vi "Copy Firmware.vi"(2 "Error In":errorcluster, 3 "Copy Software Only":bool, 4 "Image Destination":T1, 5 "Image Source":T1) -> (0 "Error Out":errorcluster, 1 "Messages":string)   [LabVIEW 2018]
uses:
  Image Parameters.ctl
  Type Defs/State Machine.ctl
  Type Defs/Global Action.ctl
  Type Defs/Save Options.ctl
  Type Defs/RT Command.ctl
  Type Defs/Insrument State.ctl
  <vilib>/nisyscfg/Set System Image (Folder).vi
  <vilib>/nisyscfg/Close (System).vi
  <vilib>/nisyscfg/Create System Image (Folder).vi
  <vilib>/nisyscfg/nisyscfg.lvlib
panel:
  out "IP Address":string
  out "Current Task":string
  # "Please wait up to a few minutes while copying firmware"
  # "(This dialog will automatically close when update is finished)"
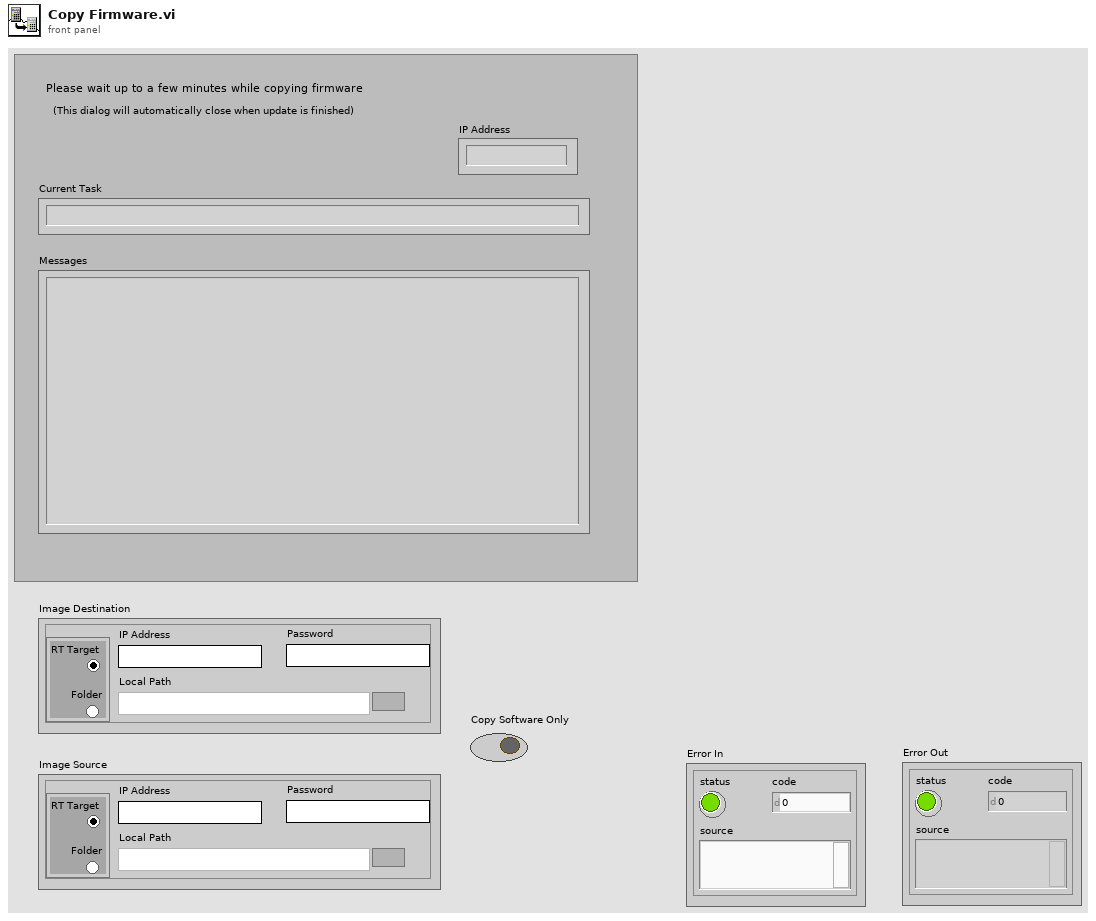
[diagram p1: front panel]
types:
  T1 = typedef "Image Parameters.ctl" = cluster{"Radio Buttons":enum32{"RT Target", "Folder"}, "Local Path":path, "IP Address":string, "Password ":string}
  T2 = typedef "State Machine.ctl" = enum16{"Wait", "Init", "Case 0", "Case 1", "Case 2", "Case 3", "Case 4", "Case 5", "Case 6", "Case 7", "Case 8", "Case 9", "Case 10", "Error", "Exit"}
  T3 = typedef "Global Action.ctl" = enum16{"Write", "Read"}
  T4 = typedef "Save Options.ctl" = enum16{"Use Dialog", "Temporary File", "My Tables", "Full Path"}
  T5 = typedef "RT Command.ctl" = enum16{"xml Start Run", "xml Start Actual Run", "xml Stop Run", "xml Runtime Update", "xml Get Status", "xml Get Table", "xml Set Table", "xml Get Configuration", "xml System Status", "xml Set LC Input Logic", "xml Get Data", "xml Get Info", "Start", "StartActualRun", "Stop", "Runtime Update", "Get Data", "Get Info", "Get Status", "Get Param", "Get Config", "Get Table", "Read ADC", "Set Oscillator", "Update Config", "Update Table", "Set All Pol", "Set Pol and DC", "Set Max Mass", "Toggle RP", "Toggle EL", "Set PIC", "Initialize Turbo", "Send Turbo Comm", "Close Turbo", "P1", "P2", "P3", "Send Serial", "Set LC Out", "Get LC In", "Read VAC", "Test Table", "Toggle Power", "Get Startup", "Set Startup", "Get ADC Table", "Set ADC Table", "Get Brief Status", "Get Detail Status", "Auxiliary Update", "Set CC Logics", "Set CC Input Logics", "Ignore Error", "invalid"}
  T6 = typedef "Insrument State.ctl" = enum16{"Initializing", "Mass Spectrometer is Off", "Starting Up", "Turning Power Off", "Going to Standby", "Roughing Pump Ready", "Turning Turbo Off", "Turbo Startup", "Turbopump Ready", "Checking Vacuum", "Going to Ready", "Ready", "Running", "Source Standby", "Lost Communication", "Shutting Down", "Fault", "24V Standby", "Go to 24V Standby", "Turbopump Ready-Waiting"}
  T7 = typedef "Global Configrations.ctl" = cluster{"Model Name":enum16{"QSight 110", "QSight 120", "QSight 210", "QSight 220", "QSight 410", "QSight 420", "IONICS 3Q 110", "IONICS 3Q 120", "IONICS 3Q 210", "IONICS 3Q 220", "IONICS 3Q 310", "IONICS 3Q 320", "Simulation (Single Source)", "Simulation (Dual Source)"}, "RunType":u16, "Acquisition State":enum16{"Ready", "Busy", "Waiting"}, "InstrState":enum16{"Initializing", "Mass Spectrometer is Off", "Starting Up", "Turning Power Off", "Going to Standby", "Roughing Pump Ready", "Turning Turbo Off", "Turbo Startup", "Turbopump Ready", "Checking Vacuum", "Going to Ready", "Ready", "Running", "Source Standby", "Lost Communication", "Shutting Down", "Fault", "24V Standby", "Go to 24V Standby", "Turbopump Ready-Waiting"}, "Run Mode":enum16{"MRM (Q1/Q2)", "Q1 Scan", "Q1 SRM", "Q2 Scan", "Q2 SRM", "Product Scan", "Precursor Scan", "Neutral Loss", "Neutral Gain"}, "Configration":T8, "TCP ID":refnum<k5>, "DT":bool, "Dead Time (nS)":i32, "Single Source":bool, "ADC Tables":T10[], "FW Udate":bool, "Simulator":bool}
  T8 = typedef "Configration.ctl" = cluster{"Table":T9[], "Instrument":string[]}
  T9 = typedef "_RT Configuration 2.ctl" = cluster{"Name":string, "Ch#":u8, "Min":dbl, "Max":dbl, "Def+":dbl, "Def-":dbl, "Offset":dbl, "Slope":dbl, "Type":u8, "Description":string, "SettleT":dbl}
  T10 = typedef "ADC Table.ctl" = cluster{"Name":string, "Ch#":u8, "Min":dbl, "Max":dbl, "Def+":dbl, "Def-":dbl, "Offset":dbl, "Slope":dbl, "Type":u8, "Description":string, "SettleT":dbl}
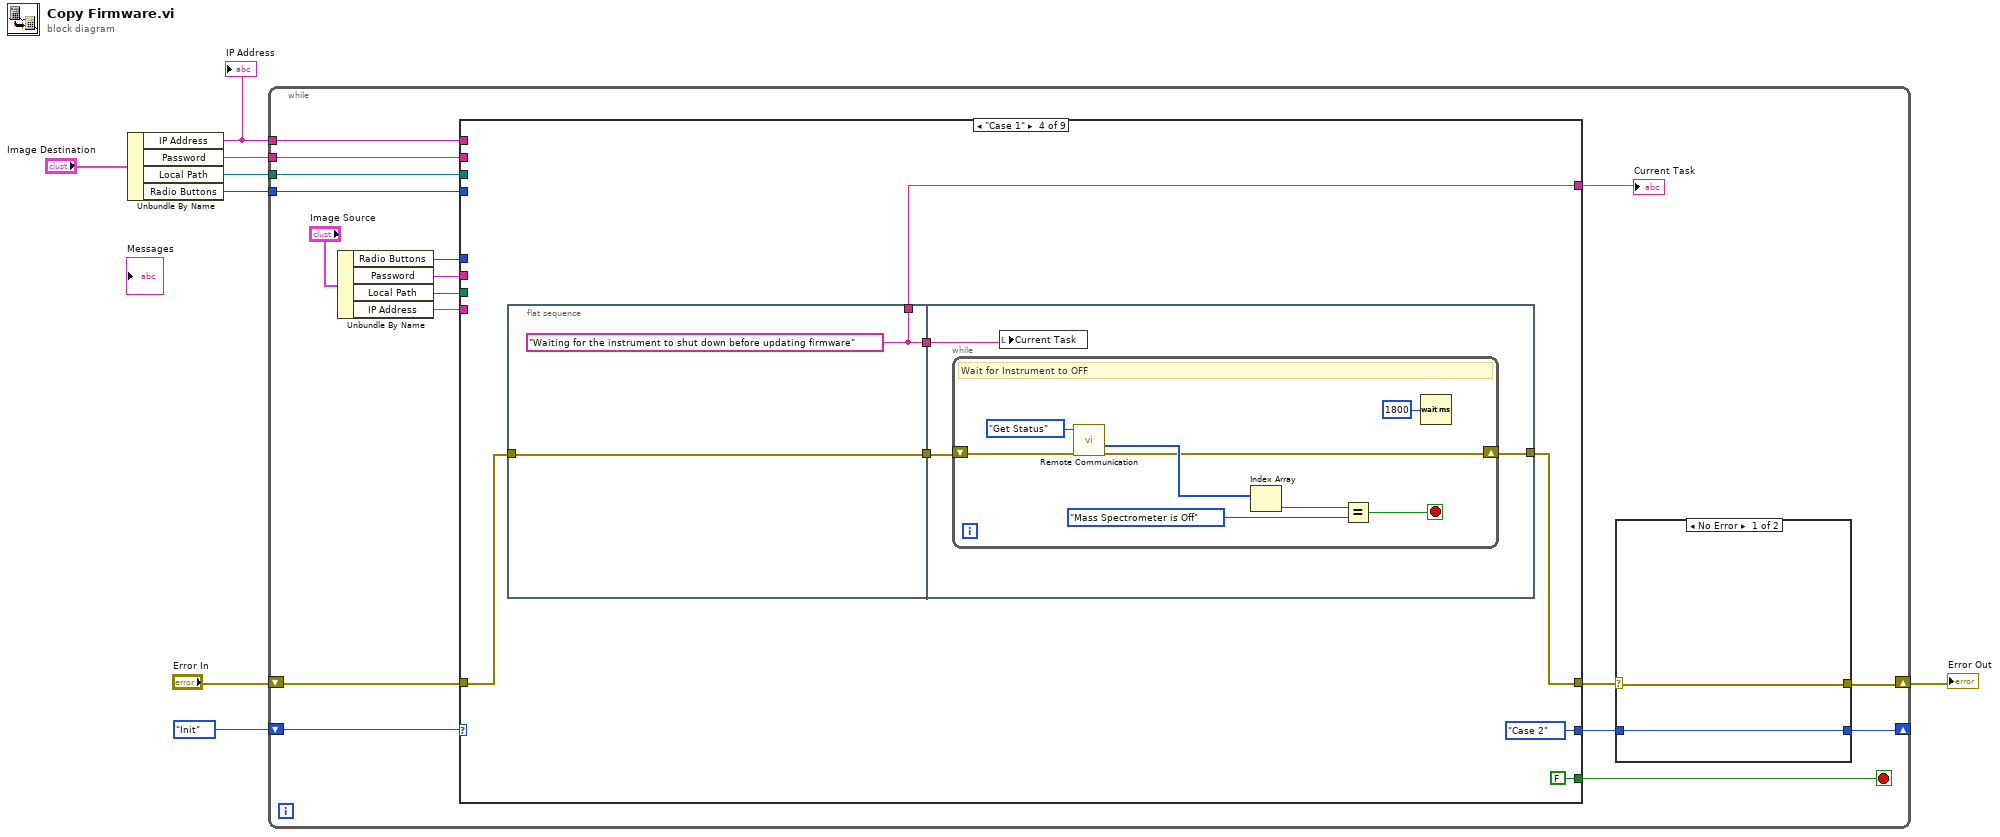
[diagram p0: block diagram]
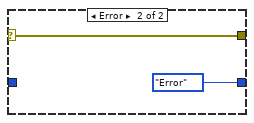
[diagram p2: hidden frame]
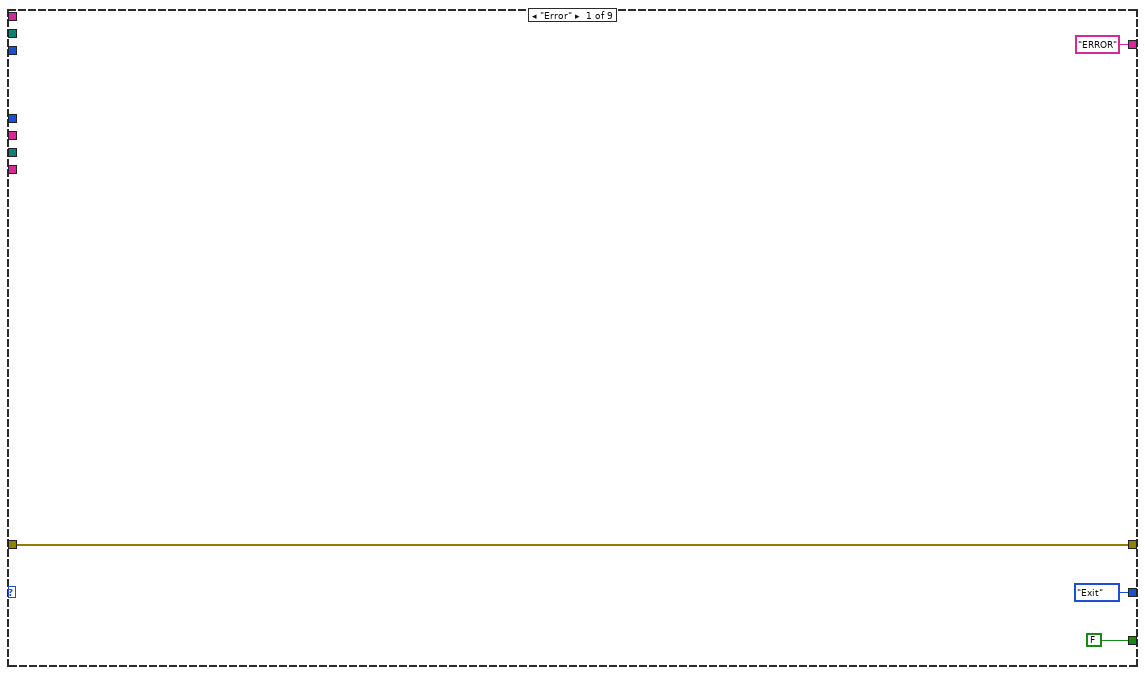
[diagram p3: hidden frame]
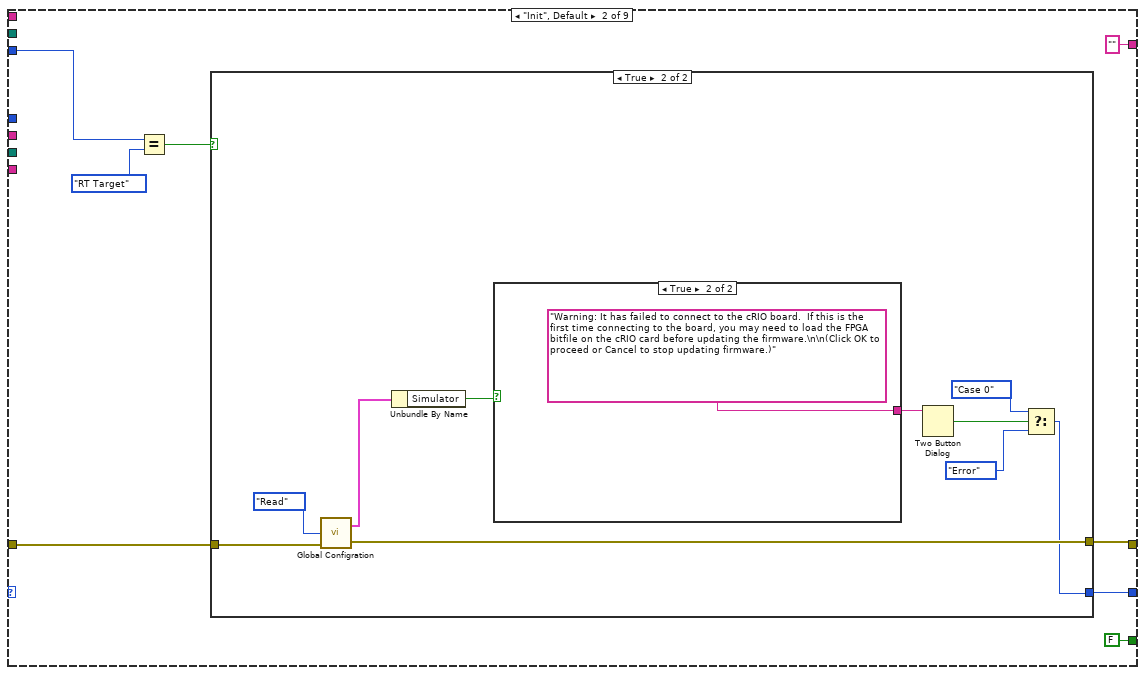
[diagram p4: hidden frame]
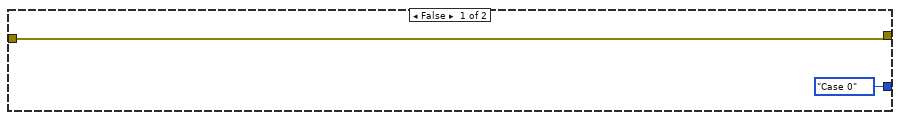
[diagram p5: hidden frame]
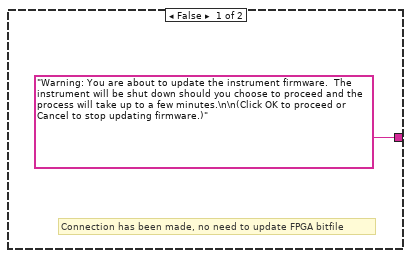
[diagram p6: hidden frame]
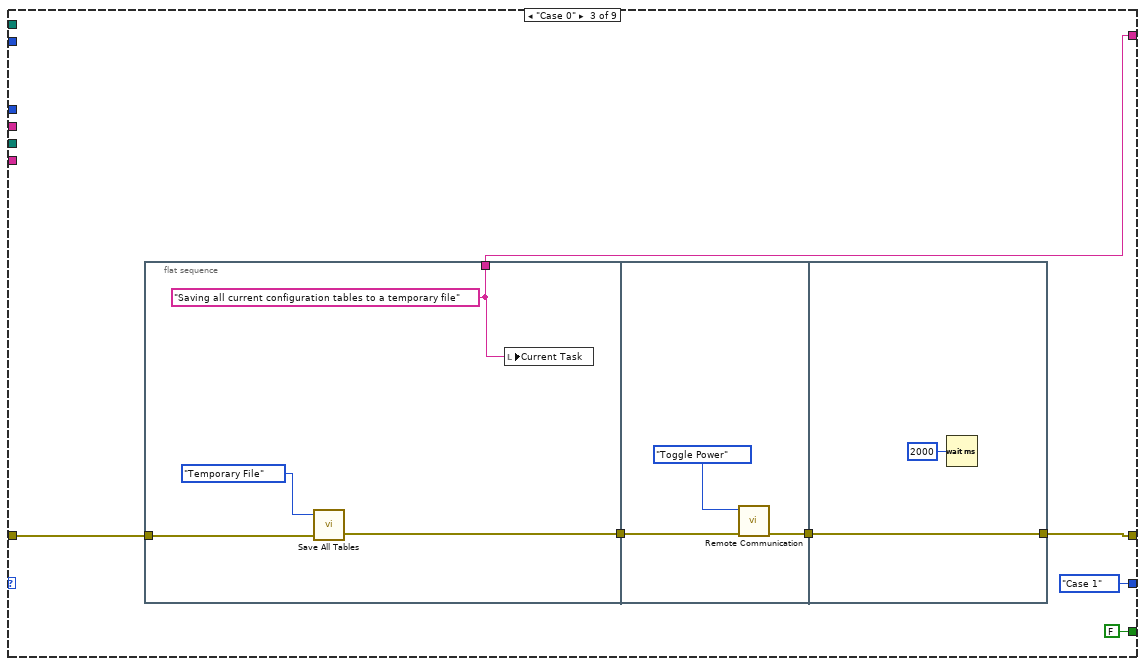
[diagram p7: hidden frame]
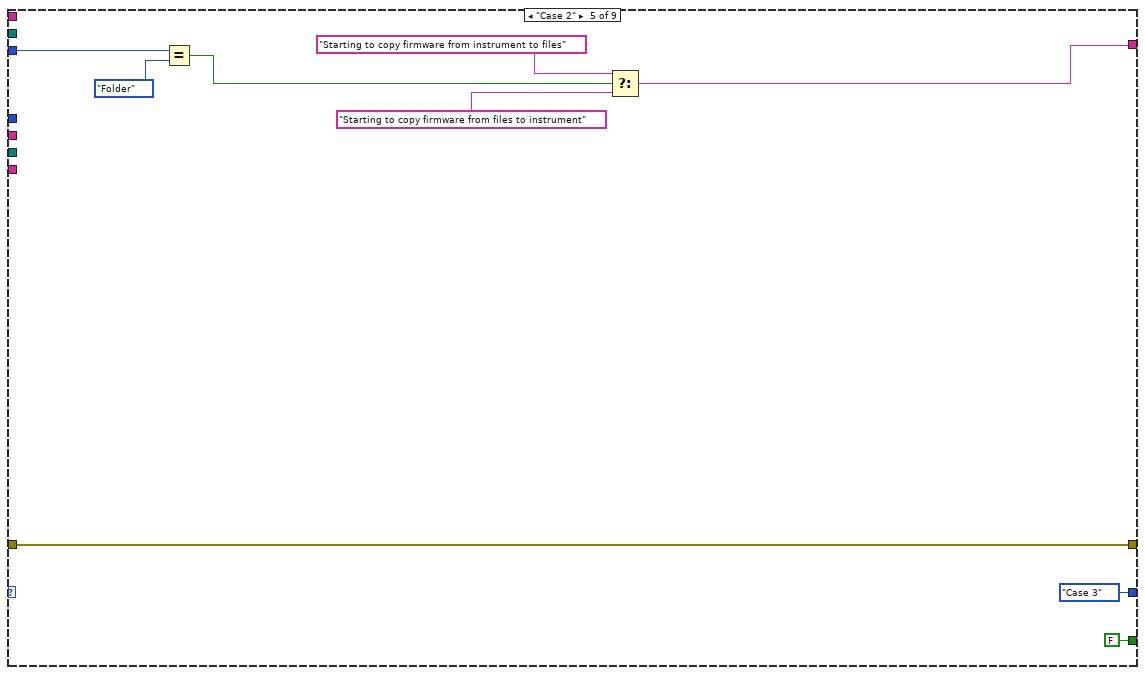
[diagram p8: hidden frame]
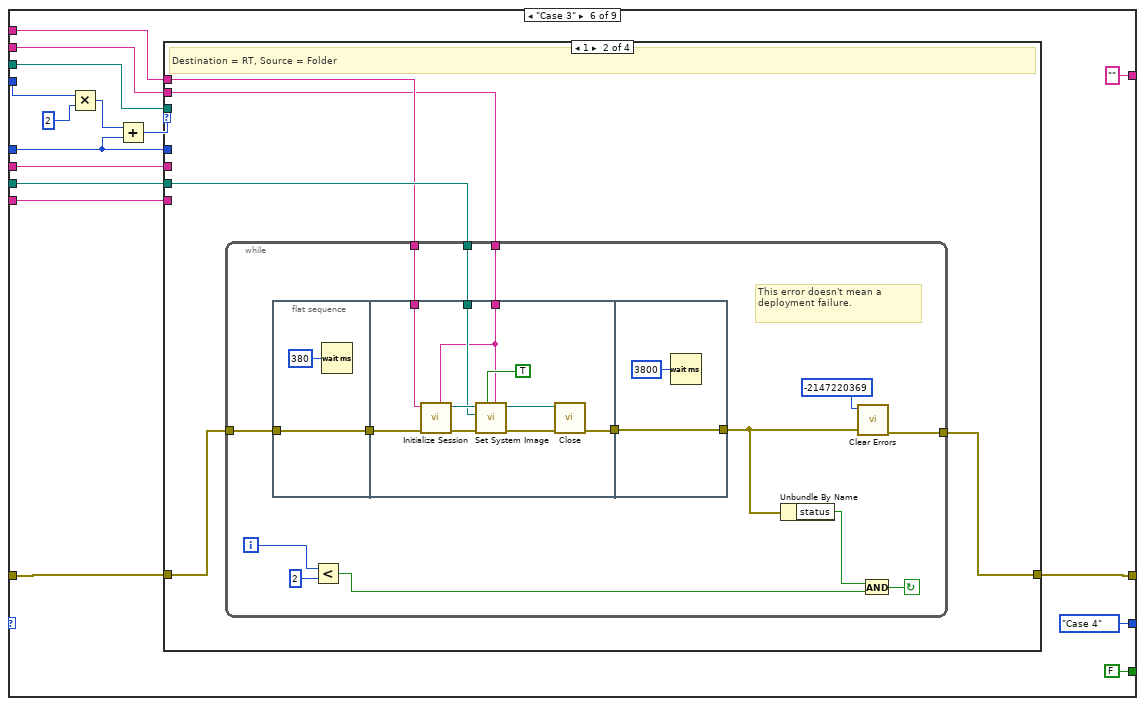
[diagram p9: hidden frame]
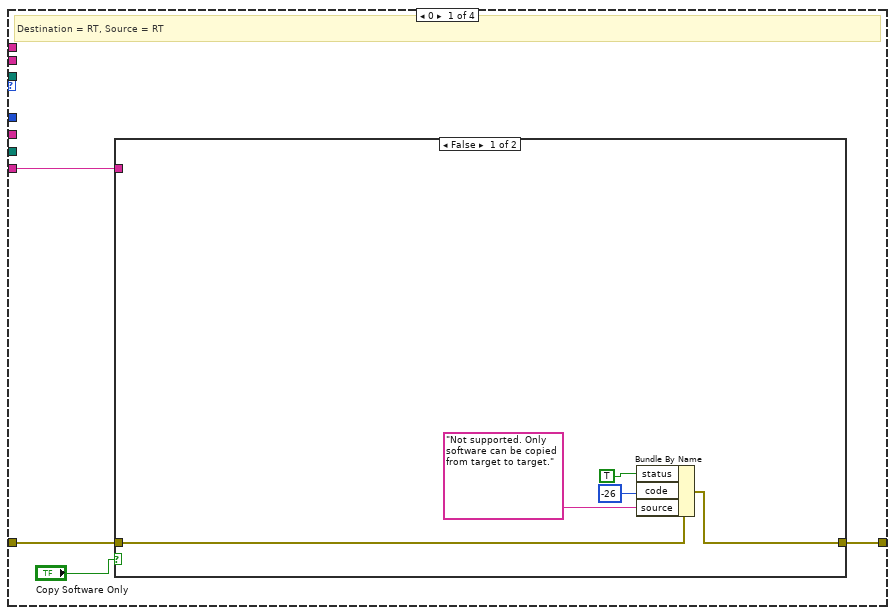
[diagram p10: hidden frame]
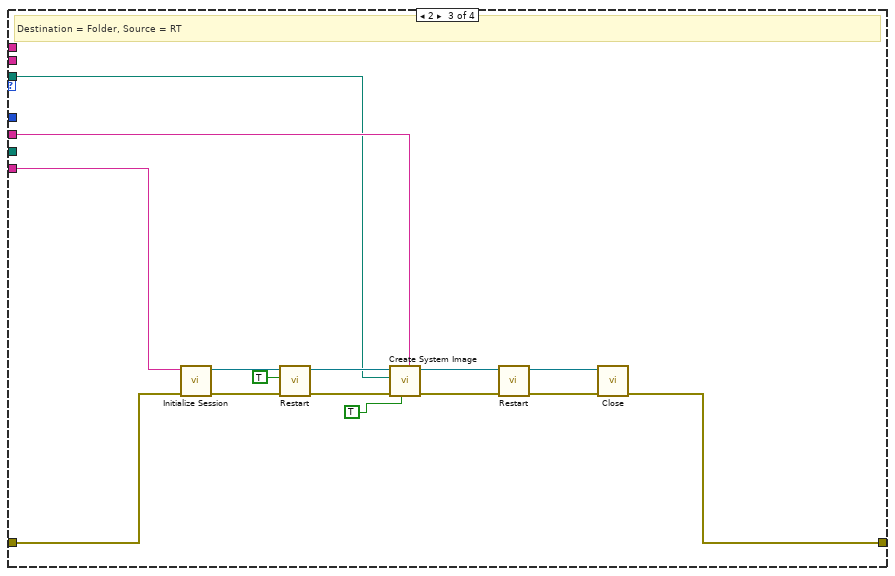
[diagram p12: hidden frame]
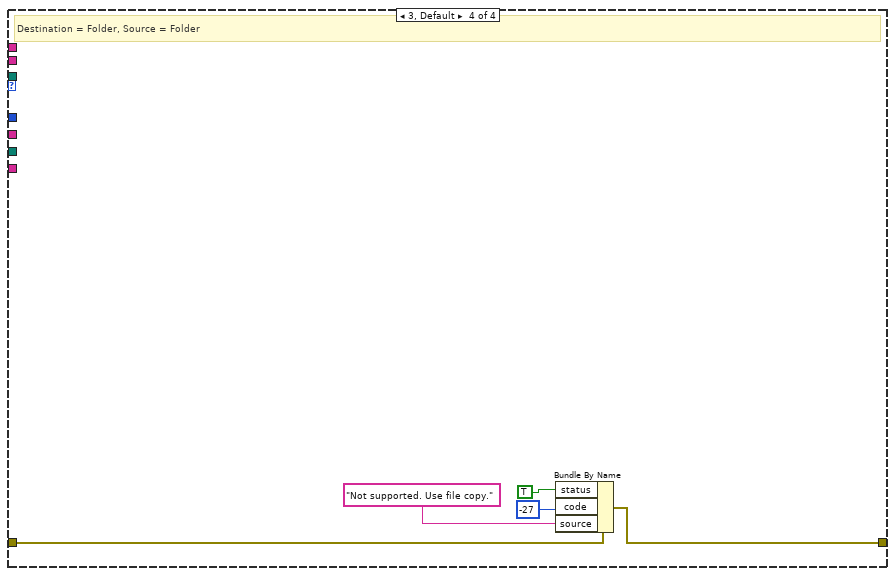
[diagram p13: hidden frame]
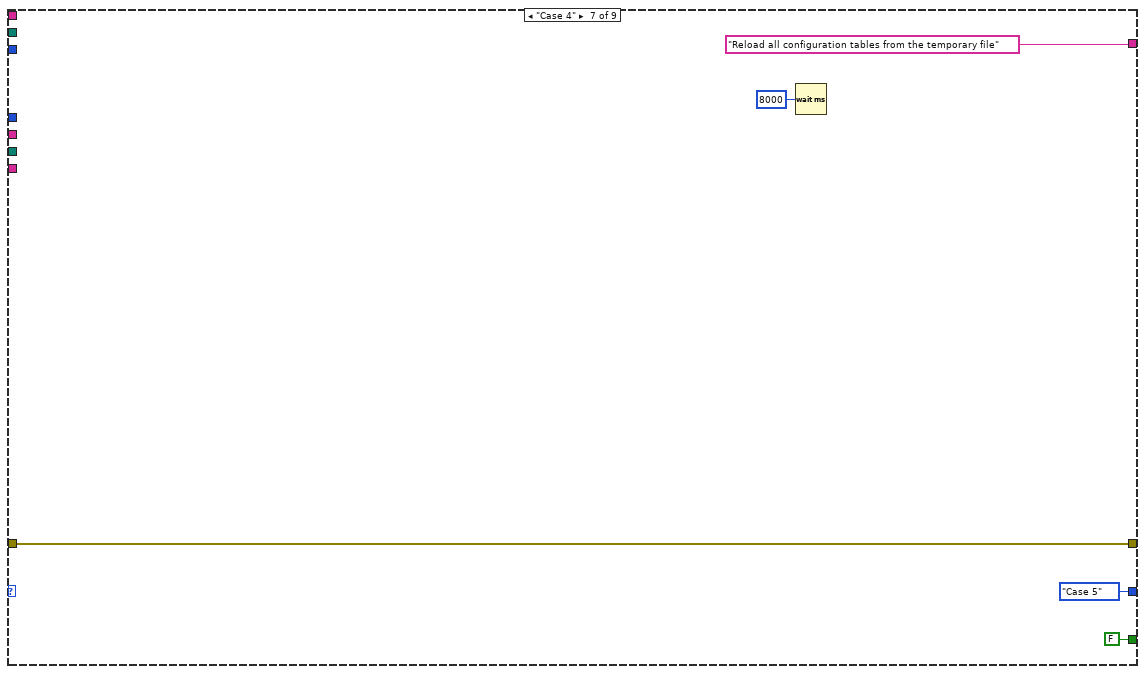
[diagram p14: hidden frame]
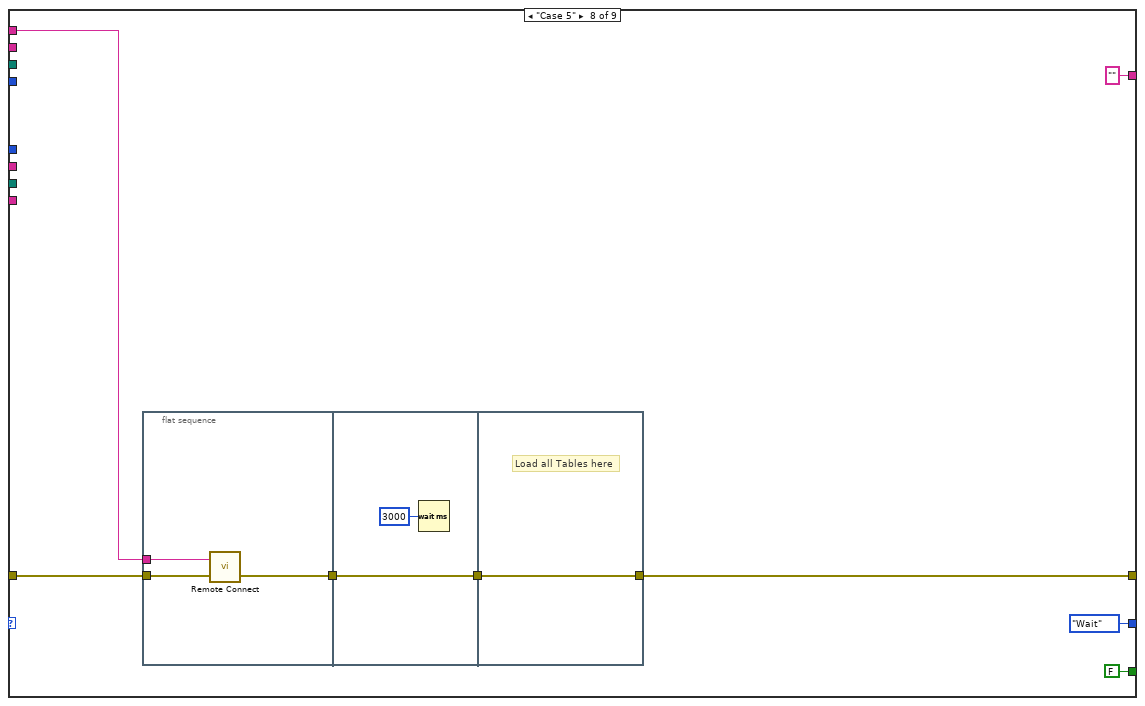
[diagram p15: hidden frame]
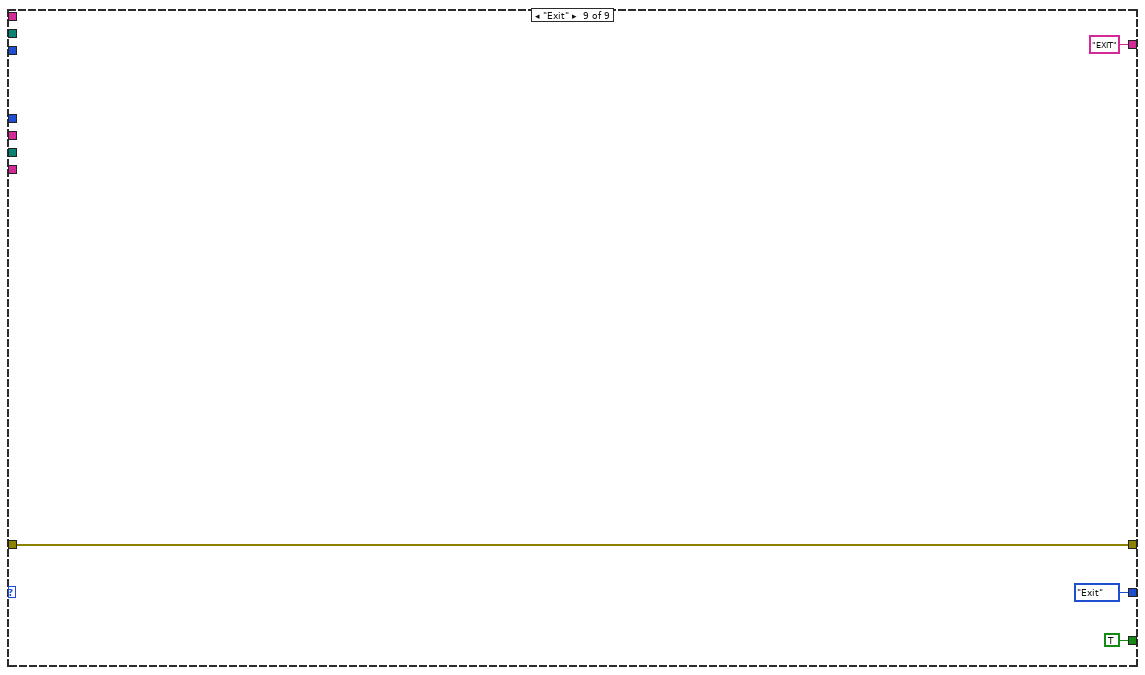
[diagram p16: hidden frame]
diagram:
  n1 = Unbundle By Name("Image Destination") -> ("IP Address"=w4:string, "Password"=w3:string, "Local Path"=w2:path, "Radio Buttons"=w1:enum32{"RT Target", "Folder"})
  "IP Address" <- w4
  n2 = while {
    shift-right: [w22] -> _
    shift-left: State_Machine."Init" ("Enum") -> [w25]
    shift-right: [w18] -> w6
    shift-left: "Error In" -> [w24]
    tunnel: w4 -> [w17]
    tunnel: w3 -> [w16]
    tunnel: w2 -> [w10]
    tunnel: w1 -> [w20]
    stop <- w9 stop-if-true
    n3 = Unbundle By Name("Image Source") -> ("Radio Buttons"=w14:enum32{"RT Target", "Folder"}, "Password"=w13:string, "Local Path"=w12:path, "IP Address"=w11:string)
    n4 = case shown="\"Case 1\"" w25 {
      tunnel: w24 -> [w30 w36 w60 w74 w94 w112 w180 w192 w200]
      tunnel: [w30 w35 w56 w73 w94 w111 w180 w188 w200] -> w23
      tunnel: [State_Machine."Exit" ("Enum") w34 State_Machine."Case 1" ("Enum") State_Machine."Case 2" ("Enum") State_Machine."Case 3" ("Enum") State_Machine."Case 4" ("Enum") State_Machine."Case 5" ("Enum") State_Machine."Wait" ("Enum") State_Machine."Exit" ("Enum")] -> w21
      tunnel: [FALSE FALSE FALSE FALSE FALSE FALSE FALSE FALSE TRUE] -> w9
      tunnel: w20 -> [_ w40 _ _ w100 w116 _ _ _]
      tunnel: ["ERROR" "" w57 w76 w95 "" "Reload all configuration tables from the temporary file" "" "EXIT"] -> w19
      tunnel: w17 -> [_ _ _ _ _ w106 _ w191 _]
      tunnel: w16 -> [_ _ _ _ _ w105 _ _ _]
      tunnel: w14 -> [_ _ _ _ _ w107 _ _ _]
      tunnel: w13 -> [_ _ _ _ _ w110 _ _ _]
      tunnel: w12 -> [_ _ _ _ _ w108 _ _ _]
      tunnel: w11 -> [_ _ _ _ _ w109 _ _ _]
      tunnel: w10 -> [_ _ _ _ _ w102 _ _ _]
      frame "Error" {
      }
      frame "Init", Default {
        n5 = Equal?(x=w40, y=enum32{"RT Target", "Folder"}."RT Target") -> (x = y?=w37:bool)
        n6 = case shown="True" w37 {
          tunnel: w36 -> [w43 w52]
          tunnel: [w43 w48] -> w35
          tunnel: [State_Machine."Case 0" ("Enum") w47] -> w34
          frame False {
          }
          frame True {
            n7 = call "Global Configration.vi"("Error In"=w52, "Action"=Global_Action."Read") -> ("Error Out"=w48:errorcluster, "Parameters Out"=w50:T7)  [unwired: 1 in]
            n8 = Unbundle By Name(w50) -> ("Simulator"=w49:bool)
            n9 = case shown="True" w49 {
              tunnel: ["Warning: You are about to update the instrument firmware.  The instrument will be shut down should you choose to proceed and the process will take up to a few minutes.\n\n(Click OK to proceed or Cancel to stop updating firmware.)" "Warning: It has failed to connect to the cRIO board.  If this is the first time connecting to the board, you may need to load the FPGA bitfile on the cRIO card before updating the firmware.\n\n(Click OK to proceed or Cancel to stop updating firmware.)"] -> w53
              frame False {
                # "Connection has been made, no need to update FPGA bitfile"
              }
              frame True {
              }
            }
            n10 = Two Button Dialog(message=w53) -> (T button?=w44:bool)  [unwired: 2 out]
            n11 = Select(t=State_Machine."Case 0" ("Enum"), s=w44, f=State_Machine."Error" ("Enum")) -> (s? t:f=w47:T2)
          }
        }
      }
      frame "Case 0" {
        n12 = flat-sequence {
          tunnel: w60 -> [w65]
          tunnel: [w64] -> w59
          tunnel: [w63] -> w57
          tunnel: w59 -> [w68]
          tunnel: [w67] -> w58
          tunnel: [w71] -> w56
          tunnel: w58 -> [w71]
          frame #0 {
            w63 = "Saving all current configuration tables to a temporary file"
            n13 = call "Save All Tables.vi"("Error In"=w65, "SaveOption(Temporary File)"=Save_Options."Temporary File") -> ("Error Out"=w64:errorcluster)  [unwired: 1 in, 1 out]
            n14 = local write "Current Task"(w63) -> ()
          }
          frame #1 {
            n15 = call "Remote Communication.vi"("Error In"=w68, "Command"=RT_Command."Toggle Power") -> ("Error Out"=w67:errorcluster)  [unwired: 4 in, 3 out]
          }
          frame #2 {
            n16 = Wait (ms)(milliseconds to wait=u32 2000) -> ()  [unwired: 1 out]
          }
        }
      }
      frame "Case 1" {
        n17 = flat-sequence {
          tunnel: [w79] -> w76
          tunnel: [w80] -> w75
          tunnel: w74 -> [w80]
          tunnel: [w79] -> w72
          tunnel: w75 -> [w83]
          tunnel: [w82] -> w73
          tunnel: w72 -> [w81]
          frame #0 {
            w79 = "Waiting for the instrument to shut down before updating firmware"
          }
          frame #1 {
            n18 = while {
              shift-right: [w86] -> w82
              shift-left: w83 -> [w85]
              stop <- w87 stop-if-true
              # "Wait for Instrument to OFF"
              n19 = call "Remote Communication.vi"("Error In"=w85, "Command"=RT_Command."Get Status") -> ("Error Out"=w86:errorcluster, "Data Array"=w90:i32[])  [unwired: 4 in, 2 out]
              n20 = Index Array(array=w90) -> (element=w91:i32)  [unwired: 1 in]
              n21 = Equal?(x=w91, y=Insrument_State."Mass Spectrometer is Off" ("InstrState")) -> (x = y?=w87:bool)
              n22 = Wait (ms)(milliseconds to wait=u32 1800) -> ()  [unwired: 1 out]
            }
            n23 = local write "Current Task"(w81) -> ()
          }
        }
      }
      frame "Case 2" {
        n24 = Equal?(x=w100, y=enum32{"RT Target", "Folder"}."Folder") -> (x = y?=w97:bool)
        n25 = Select(t="Starting to copy firmware from instrument to files", s=w97, f="Starting to copy firmware from files to instrument") -> (s? t:f=w95:string)
      }
      frame "Case 3" {
        n26 = Multiply(x=w116, y=2) -> (x*y=w114:u32)
        n27 = Add(x=w114, y=w107) -> (x+y=w113:u32)
        n28 = case shown="1" w113 {
          tunnel: w112 -> [w119 w131 w164 w176]
          tunnel: [w118 w127 w163 w175] -> w111
          tunnel: w110 -> [_ _ w162 _]
          tunnel: w109 -> [w117 _ w161 _]
          tunnel: w108 -> [_ w130 _ _]
          tunnel: w107 -> [_ _ _ _]
          tunnel: w106 -> [_ w129 _ _]
          tunnel: w105 -> [_ w128 _ _]
          tunnel: w102 -> [_ _ w160 _]
          frame 0 {
            # "Destination = RT, Source = RT"
            n29 = case shown="False" "Copy Software Only" {
              tunnel: w119 -> [w122 w126]
              tunnel: [w121 w126] -> w118
              tunnel: w117 -> [_ _]
              frame False {
                n30 = Bundle By Name(cluster=w122, "status"=TRUE, "code"=-26, "source"="Not supported. Only software can be copied from target to target.") -> (w121:errorcluster)
              }
              frame True {
              }
            }
          }
          frame 1 {
            # "Destination = RT, Source = Folder"
            n31 = while {
              tunnel: w131 -> [w145]
              tunnel: w130 -> [w135]
              tunnel: w129 -> [w134]
              tunnel: w128 -> [w133]
              tunnel: [w132] -> w127
              i -> [w140]
              stop <- w138 continue-if-true
              # "This error doesn't mean a deployment failure."
              n32 = flat-sequence {
                tunnel: w145 -> [w146]
                tunnel: [w146] -> w144
                tunnel: w144 -> [w152]
                tunnel: [w151] -> w143
                tunnel: w135 -> [w150]
                tunnel: w134 -> [w149]
                tunnel: w133 -> [w148]
                tunnel: [w159] -> w141
                tunnel: w143 -> [w159]
                frame #0 {
                  n33 = Wait (ms)(milliseconds to wait=u32 380) -> ()  [unwired: 1 out]
                }
                frame #1 {
                  n34 = call <vilib>:"Initialize Session.vi"("Password"=w148, "error in (no error)"=w152, "Target (localhost)"=w149) -> ("error out"=w154:errorcluster, "Session out"=w153:refnum<k21>)  [unwired: 7 in]
                  n35 = call-poly <vilib>:"Set System Image.vi"("Encryption Passphrase"=w148, "Restart Automatically (T)"=TRUE, "error in (no error)"=w154, "Source Folder"=w150, "Session in"=w153) -> ("error out"=w155:errorcluster, "Session out"=w156:refnum<k21>)  [unwired: 5 in]
                  n36 = call-poly <vilib>:"Close.vi"("error in (no error)"=w155, "Session in"=w156) -> ("error out"=w151:errorcluster)  [unwired: 9 in]
                }
                frame #2 {
                  n37 = Wait (ms)(milliseconds to wait=u32 3800) -> ()  [unwired: 1 out]
                }
              }
              n38 = Less?(x=w140, y=2) -> (x < y?=w136:bool)
              n39 = Unbundle By Name(w141) -> ("status"=w137:bool)
              n40 = call <vilib>:"Clear Errors.vi"("error in (no error)"=w141, "specific error code to clear (0: all)"=-2147220369) -> ("error out"=w132:errorcluster)  [unwired: 4 in, 1 out]
              n41 = And(x=w137, y=w136) -> (x .and. y?=w138:bool)
            }
          }
          frame 2 {
            # "Destination = Folder, Source = RT"
            n42 = call <vilib>:"Initialize Session.vi"("error in (no error)"=w164, "Target (localhost)"=w161) -> ("error out"=w171:errorcluster, "Session out"=w173:refnum<k21>)  [unwired: 8 in]
            n43 = call <vilib>:"Restart.vi"("error in (no error)"=w171, "Install Mode (F)"=TRUE, "Session in"=w173) -> ("error out"=w170:errorcluster, "Session out"=w172:refnum<k21>)  [unwired: 6 in, 1 out]
            n44 = call-poly <vilib>:"Create System Image.vi"("Encryption Passphrase"=w162, "Overwrite (F)"=TRUE, "error in (no error)"=w170, "Destination Folder"=w160, "Session in"=w172) -> ("error out"=w167:errorcluster, "Session out"=w168:refnum<k21>)  [unwired: 4 in, 1 out]
            n45 = call <vilib>:"Restart.vi"("error in (no error)"=w167, "Session in"=w168) -> ("error out"=w166:errorcluster, "Session out"=w165:refnum<k21>)  [unwired: 7 in, 1 out]
            n46 = call-poly <vilib>:"Close.vi"("error in (no error)"=w166, "Session in"=w165) -> ("error out"=w163:errorcluster)  [unwired: 9 in]
          }
          frame 3, Default {
            # "Destination = Folder, Source = Folder"
            n47 = Bundle By Name(cluster=w176, "status"=TRUE, "code"=-27, "source"="Not supported. Use file copy.") -> (w175:errorcluster)
          }
        }
      }
      frame "Case 4" {
        n48 = Wait (ms)(milliseconds to wait=u32 8000) -> ()  [unwired: 1 out]
      }
      frame "Case 5" {
        n49 = flat-sequence {
          tunnel: w192 -> [w195]
          tunnel: w191 -> [w194]
          tunnel: [w193] -> w190
          tunnel: w190 -> [w197]
          tunnel: [w197] -> w189
          tunnel: [w198] -> w188
          tunnel: w189 -> [w198]
          frame #0 {
            n50 = call "Remote Connect.vi"("Error In"=w195, "IP Address"=w194) -> ("Error Out"=w193:errorcluster)  [unwired: 1 out]
          }
          frame #1 {
            n51 = Wait (ms)(milliseconds to wait=u32 3000) -> ()  [unwired: 1 out]
          }
          frame #2 {
            # "Load all Tables here"
          }
        }
      }
      frame "Exit" {
      }
    }
    "Current Task" <- w19
    n52 = case shown="No Error" w23 {
      selector: w23 -> [w26 w28]
      tunnel: [w27 State_Machine."Error" ("Enum")] -> w22
      tunnel: w21 -> [w27 _]
      tunnel: [w26 w28] -> w18
      frame No Error {
      }
      frame Error {
      }
    }
  }
  "Error Out" <- w6
